vi "ReadPulsePositions.vi"(8 "error in (no error)":errorcluster, 11 "Map":T2) -> (0 "error out":errorcluster, 2 "found":bool, 3 "pulse positions array":T1[](array[typedef]))   [LabVIEW 2017]
uses:
  <vilib>/addons/PointValueMap/controls/PointMap.ctl
  <vilib>/addons/InsightCM/Utilities/Analysis/Shared/controls/PulsePositions.ctl
  <vilib>/addons/PointValueMap/subVIs/Point_Read_variant.vi
  <vilib>/addons/PointValueMap/PointValueMap.lvlib
  <vilib>/addons/InsightCM/Utilities/Analysis/Shared/AnalysisHelper.lvlib
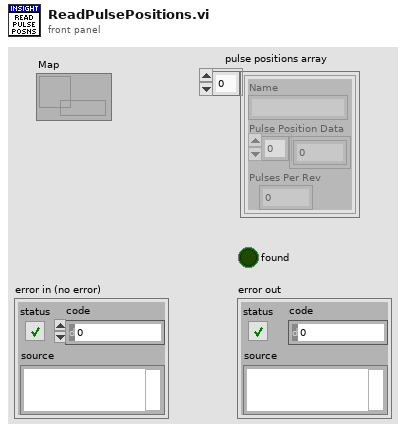
[diagram p1: front panel]
types:
  T1 = typedef "AnalysisHelper.lvlib/PulsePositions.ctl" = cluster{"Name":string, "Pulse Position Data":dbl[], "Pulses Per Rev":i32}
  T2 = typedef "PointValueMap.lvlib/PointMap.ctl" = refnum<data-value>
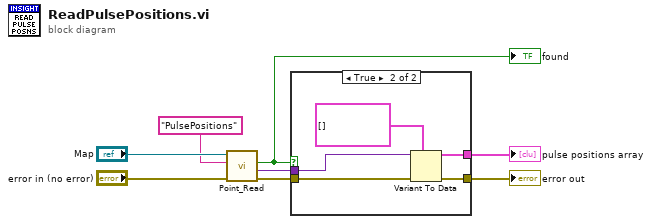
[diagram p0: block diagram]
diagram:
  n1 = call-poly <vilib>:"Point_Read.vi"("Error In"="error in (no error)", "Tag"="PulsePositions", "Map"="Map") -> ("Error Out"=w6:errorcluster, "Value"=w7:variant, "Found?"=w3:bool)  [unwired: 3 in, 3 out]
  "found" <- w3
  n2 = case shown="True" w3 {
    tunnel: [w9 w14] -> w8
    tunnel: w7 -> [_ w13]
    tunnel: w6 -> [w9 w12]
    tunnel: [_ w11] -> w1
    frame False {
    }
    frame True {
      n3 = Variant To Data(error in=w12, type=T1[] [] ("pulse positions array"), Variant=w13) -> (data=w11:T1[], error out=w14:errorcluster)
    }
  }
  "error out" <- w8
  "pulse positions array" <- w1
